vi "FrontEnd_Module.vi"() -> ()   [LabVIEW 2023]
uses:
  Controls/Select_Preference.ctl
  Controls/Coffee_Machine_Dispaly.ctl
  Controls/Queue_Operation_Select.ctl
  Controls/Coffee_Machine_Data.ctl
  Controls/Quantity_Data.ctl
  Controls/State_and_Data.ctl
  Controls/File_Operation_Select.ctl
  <vilib>/Utility/file.llb/Read Delimited Spreadsheet (string).vi
panel:
  out "Error_Out":errorcluster
  in  "Error_In":errorcluster
  in  "Power":bool
  out "Dispaly":T1 {"Dispenser" scale=0.0..80.0; "Chamber" scale=0.0..80.0}
  in  "Selector":T2 {"Select_Bevarage" scale=0.0..2.0}
  # "Coffee"
  # "Latte"
  # "Hot Water"
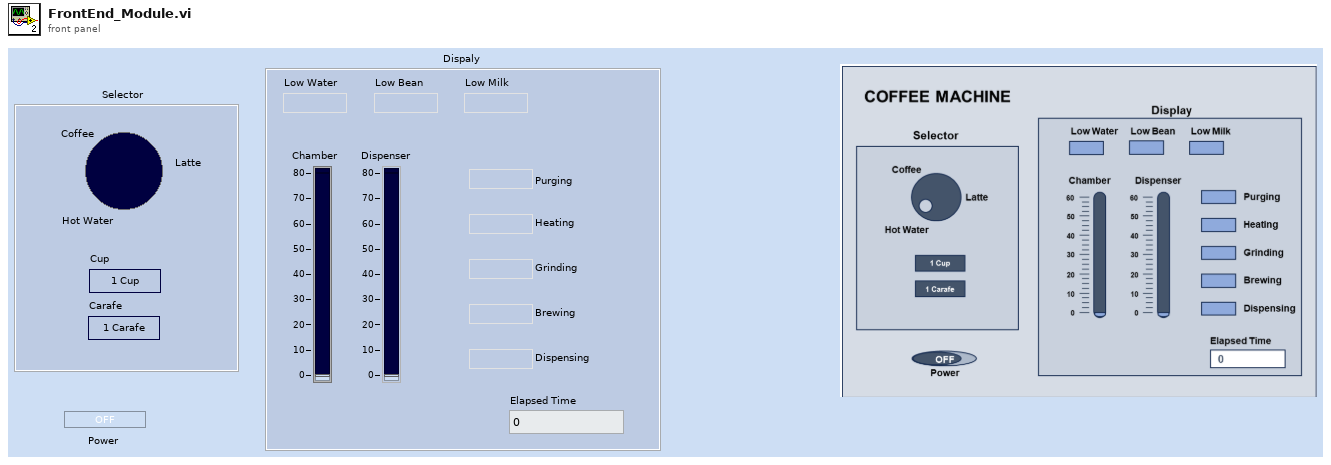
[diagram p1: front panel]
types:
  T1 = typedef "Coffee_Machine_Dispaly.ctl" = cluster{"Low_Water":bool, "Low_Bean":bool, "Low_Milk":bool, "Chamber":dbl, "Dispenser":dbl, "Purging":bool, "Heating":bool, "Grinding":bool, "Brewing":bool, "Dispensing":bool, "Elapsed_Time":dbl}
  T2 = typedef "Select_Preference.ctl" = cluster{"Select_Bevarage":i32, "Cup":bool, "Carafe":bool}
  T3 = typedef "State_and_Data.ctl" = cluster{"State":string, "Data":variant}
  T4 = typedef "Queue_Operation_Select.ctl" = enum16{"Obtain_Queue", "Enqueue", "Enqueue_First", "Enqueue_N", "Lossy_Enqueue", "Preview", "Queue_Status", "Dequeue", "Flush", "Release_Queue"}
  T5 = typedef "Coffee_Machine_Data.ctl" = cluster{"Backend_Data":T6, "Selector":T2, "Cup_Unit":dbl, "Carafe_Unit":dbl, "Ingreedient_File_PAth":path, "Process_Needed":string[], "Indredient_Needed":string[], "Time_Needed":string[], "State_and_Data":T3, "Chamber_Quantity":dbl, "Dispenser_Quantiry":dbl, "Dispaly":T1}
  T6 = typedef "Quantity_Data.ctl" = cluster{"Level":cluster{"Water_Level":dbl, "Bean_Level":dbl, "Milk_Level":dbl}, "Total_Cups":dbl}
  T7 = cluster{"Water_Level":dbl, "Bean_Level":dbl, "Milk_Level":dbl}
  T8 = typedef "File_Operation_Select.ctl" = enum16{"Open", "Read", "Write", "Close"}
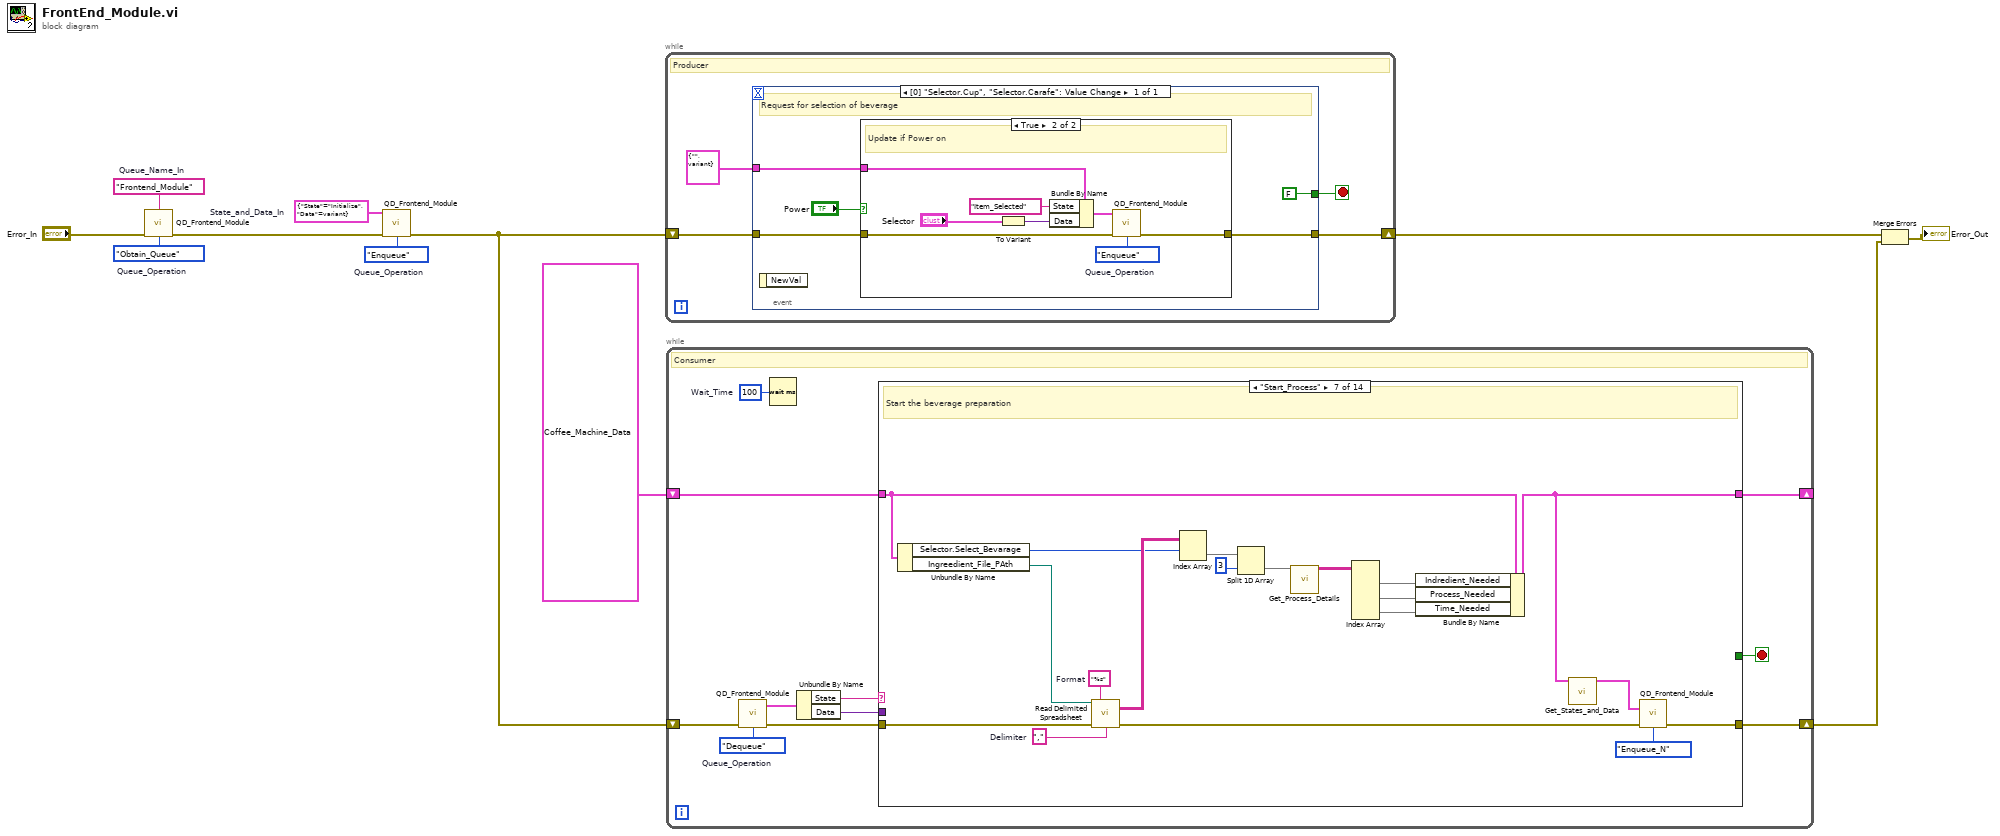
[diagram p0: block diagram]
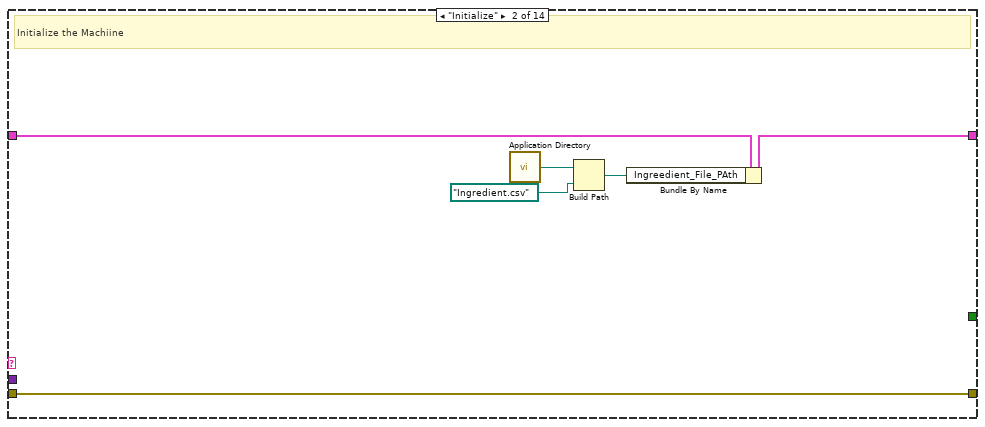
[diagram p3: hidden frame]
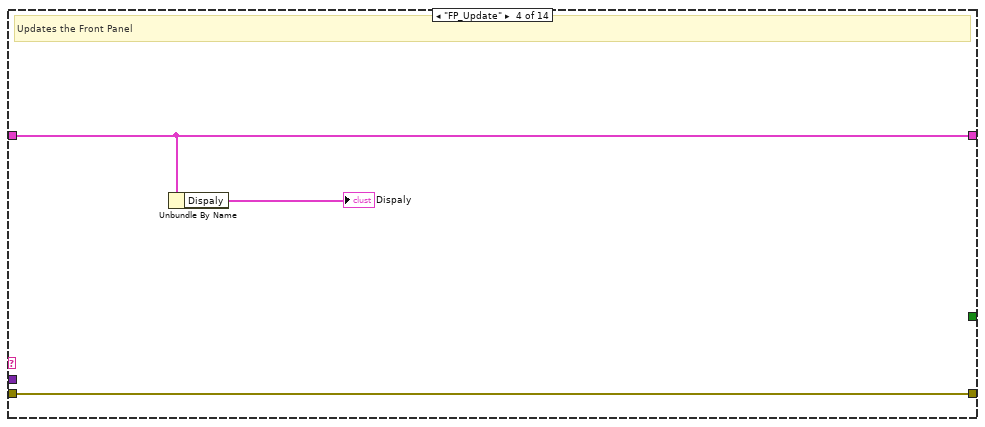
[diagram p5: hidden frame]
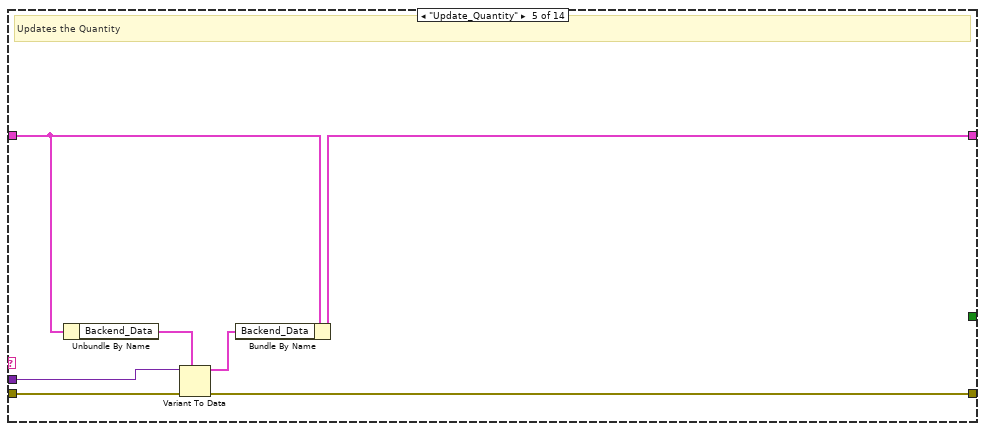
[diagram p6: hidden frame]
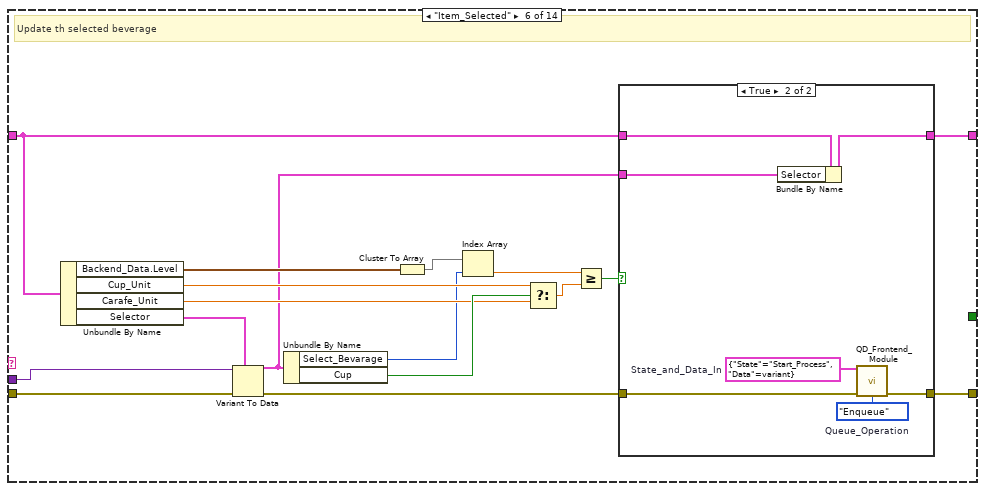
[diagram p7: hidden frame]
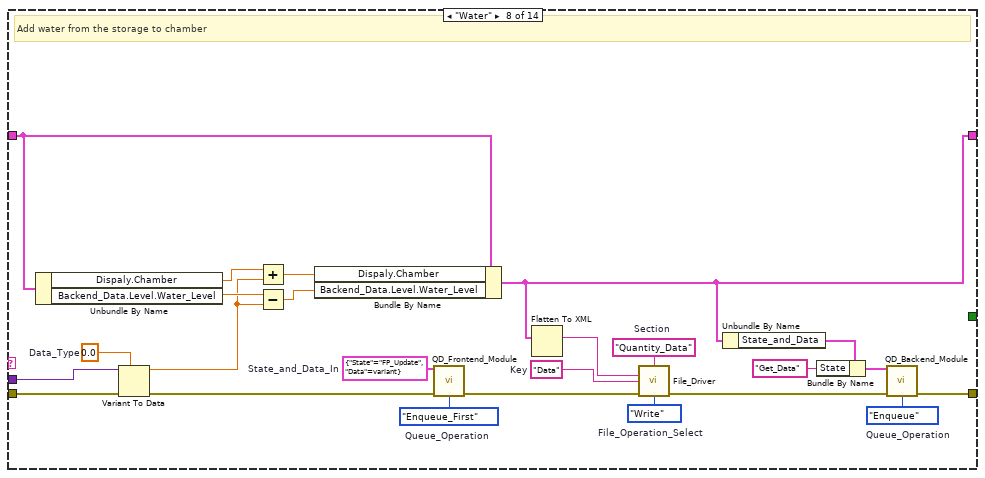
[diagram p9: hidden frame]
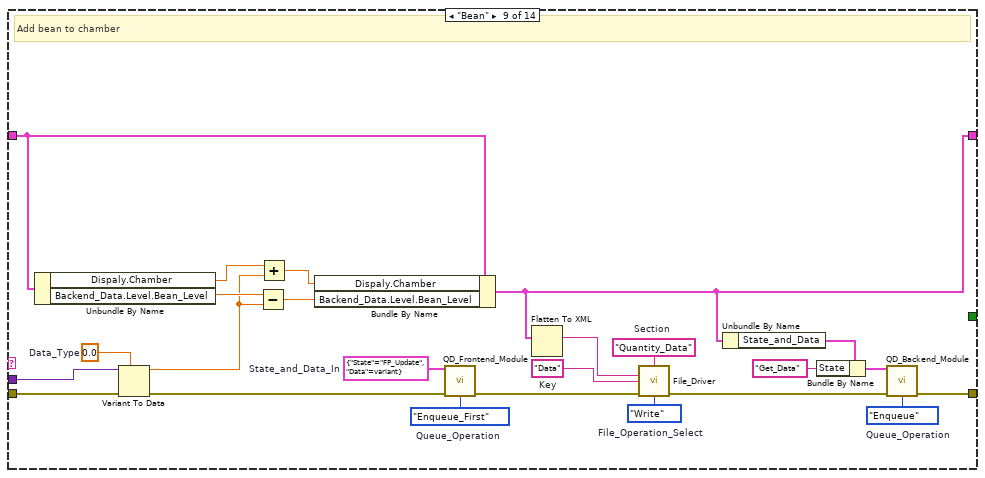
[diagram p10: hidden frame]
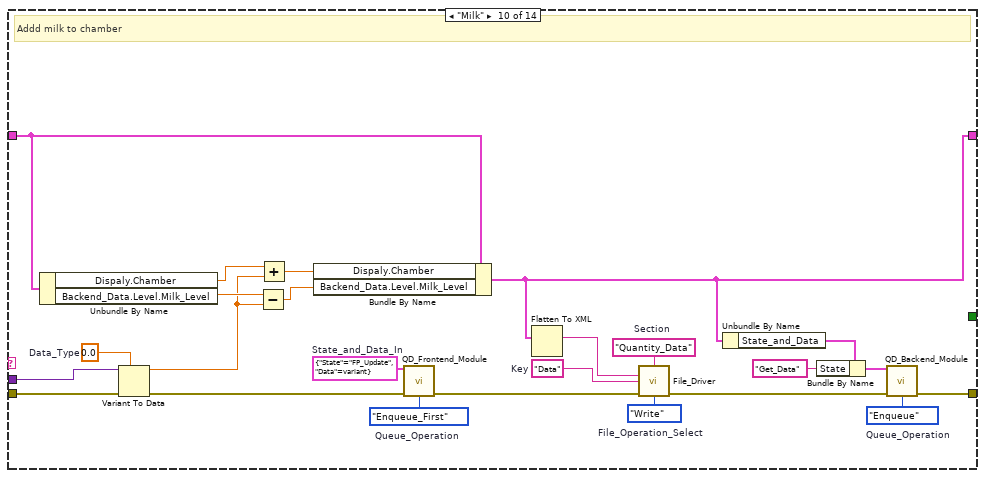
[diagram p11: hidden frame]
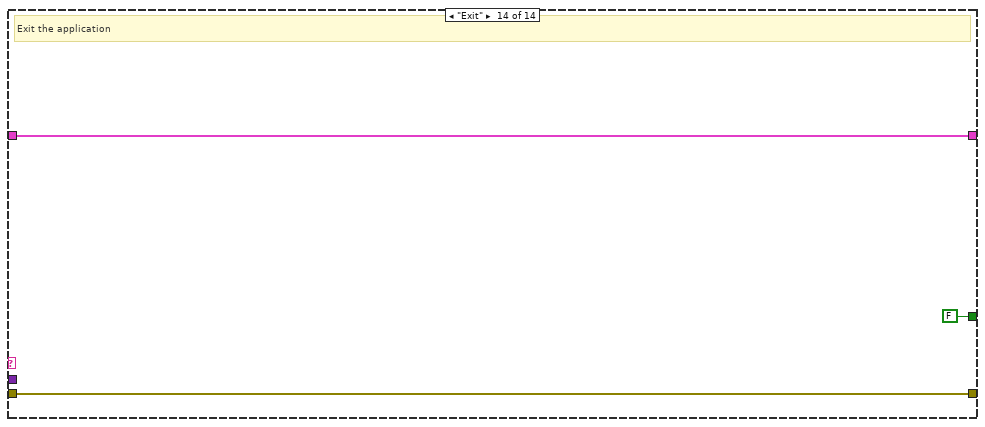
[diagram p15: hidden frame]
diagram:
  w1 = T3 {"State"="Initialize", "Data"=variant}  # State_and_Data_In
  w2 = Queue_Operation_Select."Enqueue"  # Queue_Operation
  w9 = "Frontend_Module"  # Queue_Name_In
  w10 = Queue_Operation_Select."Obtain_Queue"  # Queue_Operation
  n1 = call "QD_Frontend_Module.vi"("Queue_Name_In"=w9, "Error_In"="Error_In", "Queue_Operation"=w10) -> ("Error_Out"=w7:errorcluster)  [unwired: 10 in, 2 out]
  n2 = call "QD_Frontend_Module.vi"("State_and_Data_In"=w1, "Error_In"=w7, "Queue_Operation"=w2) -> ("Error_Out"=w3:errorcluster)  [unwired: 10 in, 2 out]
  n3 = while {
    shift-right: [w15] -> w8
    shift-left: w3 -> [w14]
    stop <- w12 stop-if-true
    # "Producer"
    n4 = event shown="[0] \"Selector.Cup\", \"Selector.Carafe\": Value Change" {
      selector: _ -> [_]
      dyn-events: _ -> [_]
      timeout: _ -> [_]
      tunnel: [w19] -> w15
      tunnel: w14 -> [w20]
      tunnel: T3 {"State"="", "Data"=variant} ("State_and_Data") -> [w18]
      tunnel: [FALSE] -> w12
      event Value Change {
        # "Request for selection of beverage"
        n5 = event-data() -> ()  [unwired: 1 in, 1 out]
        n6 = case shown="True" "Power" {
          tunnel: w20 -> [w21 w29]
          tunnel: [w21 w28] -> w19
          tunnel: w18 -> [_ w23]
          frame False {
          }
          frame True {
            w27 = Queue_Operation_Select."Enqueue"  # Queue_Operation
            # "Update if Power on"
            n7 = To Variant(anything="Selector") -> (Variant=w25:variant)
            n8 = Bundle By Name(cluster=w23, "State"="Item_Selected", "Data"=w25) -> (w24:T3)
            n9 = call "QD_Frontend_Module.vi"("State_and_Data_In"=w24, "Error_In"=w29, "Queue_Operation"=w27) -> ("Error_Out"=w28:errorcluster)  [unwired: 10 in, 2 out]
          }
        }
      }
    }
  }
  n10 = while {
    shift-right: [w32] -> _
    shift-left: T5 {"Backend_Data"={"Level"={"Water_Level"=0.0, "Bean_Level"=0.0, "Milk_Level"=0.0}, "Total_Cups"=0.0}, "Selector"={"Select_Bevarage"=0, "Cup"=FALSE, "Carafe"=FALSE}, "Cup_Unit"=5.0, "Carafe_Unit"=20.0, "Ingreedient_File_PAth"=path "", "Process_Needed"=[], "Indredient_Needed"=[], "Time_Needed"=[], "State_and_Data"={"State"="", "Data"=variant}, "Chamber_Quantity"=0.0, "Dispenser_Quantiry"=0.0, "Dispaly"={"Low_Water"=FALSE, "Low_Bean"=FALSE, "Low_Milk"=FALSE, "Chamber"=0.0, "Dispenser"=0.0, "Purging"=FALSE, "Heating"=FALSE, "Grinding"=FALSE, "Brewing"=FALSE, "Dispensing"=FALSE, "Elapsed_Time"=0.0}} -> [w33]
    shift-right: [w34] -> w4
    shift-left: w3 -> [w40]
    stop <- w31 stop-if-true
    w30 = u32 100  # Wait_Time
    w38 = Queue_Operation_Select."Dequeue"  # Queue_Operation
    # "Consumer"
    n11 = call "QD_Frontend_Module.vi"("Error_In"=w40, "Queue_Operation"=w38) -> ("State_and_Data_Out"=w37:T3, "Error_Out"=w39:errorcluster)  [unwired: 11 in, 1 out]
    n12 = Wait (ms)(milliseconds to wait=w30) -> ()  [unwired: 1 out]
    n13 = Unbundle By Name(w37) -> ("State"=w36:string, "Data"=w35:variant)
    n14 = case shown="\"Start_Process\"" w36 {
      tunnel: w39 -> [w42 w48 w50 w53 w60 w77 w105 w129 w153 w177 w179 w181 w183 w186]
      tunnel: w35 -> [_ _ _ _ w58 w76 _ w127 w152 w176 _ _ _ _]
      tunnel: [w42 w48 w50 w53 w59 w70 w93 w122 w147 w171 w179 w181 w183 w186] -> w34
      tunnel: w33 -> [w41 w47 w49 w52 w57 w63 w89 w125 w150 w174 w178 w180 w182 w185]
      tunnel: [w41 w46 w49 w52 w55 w64 w88 w115 w140 w164 w178 w180 w182 w185] -> w32
      tunnel: [_ _ _ _ _ _ _ _ _ _ _ _ _ FALSE] -> w31
      frame Default {
      }
      frame "Initialize" {
        # "Initialize the Machiine"
        n15 = call <vilib>:"Application Directory.vi"() -> ("Application Directory"=w44:path)
        n16 = Build Path(base path=w44, name or relative path=path "Ingredient.csv" ("Ingreedient_File_PAth")) -> (appended path=w45:path)
        n17 = Bundle By Name(cluster=w47, "Ingreedient_File_PAth"=w45) -> (w46:T5)
      }
      frame "Disable_and_Enable" {
        # "Disaable and enable"
      }
      frame "FP_Update" {
        # "Updates the Front Panel"
        n18 = Unbundle By Name(w52) -> ("Dispaly"=→"Dispaly":T1)
      }
      frame "Update_Quantity" {
        # "Updates the Quantity"
        n19 = Unbundle By Name(w57) -> ("Backend_Data"=w56:T6)
        n20 = Variant To Data(error in=w60, type=w56, Variant=w58) -> (data=w54:T6, error out=w59:errorcluster)
        n21 = Bundle By Name(cluster=w57, "Backend_Data"=w54) -> (w55:T5)
      }
      frame "Item_Selected" {
        # "Update th selected beverage"
        n22 = Unbundle By Name(w63) -> ("Backend_Data.Level"=w68:T7, "Cup_Unit"=w74:dbl, "Carafe_Unit"=w73:dbl, "Selector"=w62:T2)
        n23 = Variant To Data(error in=w77, type=w62, Variant=w76) -> (data=w61:T2, error out=w69:errorcluster)
        n24 = Unbundle By Name(w61) -> ("Select_Bevarage"=w66:i32, "Cup"=w75:bool)
        n25 = Cluster To Array(cluster=w68) -> (array=w67:dbl[])
        n26 = Index Array(array=w67, index=w66) -> (element=w65:dbl)
        n27 = Select(t=w74, s=w75, f=w73) -> (s? t:f=w71:dbl)
        n28 = Greater Or Equal?(x=w65, y=w71) -> (x >= y?=w72:bool)
        n29 = case shown="True" w72 {
          tunnel: [w78 w82] -> w70
          tunnel: w69 -> [w78 w86]
          tunnel: [w79 w84] -> w64
          tunnel: w63 -> [w79 w85]
          tunnel: w61 -> [_ w83]
          frame False {
          }
          frame True {
            w80 = T3 {"State"="Start_Process", "Data"=variant}  # State_and_Data_In
            w81 = Queue_Operation_Select."Enqueue"  # Queue_Operation
            n30 = Bundle By Name(cluster=w85, "Selector"=w83) -> (w84:T5)
            n31 = call "QD_Frontend_Module.vi"("State_and_Data_In"=w80, "Error_In"=w86, "Queue_Operation"=w81) -> ("Error_Out"=w82:errorcluster)  [unwired: 10 in, 2 out]
          }
        }
      }
      frame "Start_Process" {
        w102 = "%s"  # Format
        w103 = ","  # Delimiter
        # "Start the beverage preparation"
        n32 = Unbundle By Name(w89) -> ("Selector.Select_Bevarage"=w100:i32, "Ingreedient_File_PAth"=w87:path)
        n33 = call-poly <vilib>:"Read Delimited Spreadsheet.vi"("file path (dialog if empty)"=w87, "format (%s)"=w102, "error in (no error)"=w105, "delimiter (\\t)"=w103) -> ("all rows"=w101:string[][], "error out"=w104:errorcluster)  [unwired: 6 in, 4 out]
        n34 = Index Array(array=w101, index (row)=w100) -> (element=w99:string[])  [unwired: 1 in]
        n35 = Split 1D Array(array=w99, index=3) -> (second subarray=w97:string[])  [unwired: 1 out]
        n36 = call "Get_Process_Details.vi"("Process_Data"=w97) -> ("Needs"=w96:string[][])  [unwired: 14 in]
        n37 = Index Array(array=w96) -> (element #1=w91:string[], element #2=w95:string[], element #3=w94:string[])  [unwired: 6 in]
        n38 = Bundle By Name(cluster=w89, "Indredient_Needed"=w91, "Process_Needed"=w95, "Time_Needed"=w94) -> (w88:T5)
        n39 = call "Get_States_and_Data.vi"("Coffee_Machine_Data"=w88) -> ("States_and_Data"=w90:T3[])  [unwired: 14 in]
        n40 = call "QD_Frontend_Module.vi"("State_and_Data_N_In"=w90, "Error_In"=w104, "Queue_Operation"=Queue_Operation_Select."Enqueue_N") -> ("Error_Out"=w93:errorcluster)  [unwired: 10 in, 2 out]
      }
      frame "Water" {
        w106 = Queue_Operation_Select."Enqueue_First"  # Queue_Operation
        w107 = T3 {"State"="FP_Update", "Data"=variant}  # State_and_Data_In
        w112 = "Quantity_Data"  # Section
        w113 = "Data"  # Key
        w116 = File_Operation_Select."Write"  # File_Operation_Select
        w121 = Queue_Operation_Select."Enqueue"  # Queue_Operation
        w126 = 0.0  # Data_Type
        # "Add water from the storage to chamber"
        n41 = Unbundle By Name(w125) -> ("Dispaly.Chamber"=w109:dbl, "Backend_Data.Level.Water_Level"=w124:dbl)
        n42 = Variant To Data(error in=w129, type=w126, Variant=w127) -> (data=w110:dbl, error out=w128:errorcluster)
        n43 = Add(x=w109, y=w110) -> (x+y=w111:dbl)
        n44 = Subtract(x=w124, y=w110) -> (x-y=w123:dbl)
        n45 = Bundle By Name(cluster=w125, "Dispaly.Chamber"=w111, "Backend_Data.Level.Water_Level"=w123) -> (w115:T5)
        n46 = call "QD_Frontend_Module.vi"("State_and_Data_In"=w107, "Error_In"=w128, "Queue_Operation"=w106) -> ("Error_Out"=w108:errorcluster)  [unwired: 10 in, 2 out]
        n47 = Flatten To XML(6:w115) -> (2:w114:string)
        n48 = call "File_Driver.vi"("Section"=w112, "Data_In"=w114, "Key"=w113, "Error_In"=w108, "File_Operation_Select"=w116) -> ("Error_Out"=w117:errorcluster)  [unwired: 9 in, 1 out]
        n49 = Unbundle By Name(w115) -> ("State_and_Data"=w119:T3)
        n50 = Bundle By Name(cluster=w119, "State"="Get_Data") -> (w120:T3)
        n51 = call "QD_Backend_Module.vi"("State_and_Data_In"=w120, "Error_In"=w117, "Queue_Operation"=w121) -> ("Error_Out"=w122:errorcluster)  [unwired: 10 in, 2 out]
      }
      frame "Bean" {
        w135 = Queue_Operation_Select."Enqueue_First"  # Queue_Operation
        w136 = T3 {"State"="FP_Update", "Data"=variant}  # State_and_Data_In
        w137 = "Quantity_Data"  # Section
        w138 = "Data"  # Key
        w141 = File_Operation_Select."Write"  # File_Operation_Select
        w146 = Queue_Operation_Select."Enqueue"  # Queue_Operation
        w151 = 0.0  # Data_Type
        # "Add bean to chamber"
        n52 = Unbundle By Name(w150) -> ("Dispaly.Chamber"=w132:dbl, "Backend_Data.Level.Bean_Level"=w149:dbl)
        n53 = Variant To Data(error in=w153, type=w151, Variant=w152) -> (data=w131:dbl, error out=w134:errorcluster)
        n54 = Subtract(x=w149, y=w131) -> (x-y=w148:dbl)
        n55 = Add(x=w132, y=w131) -> (x+y=w130:dbl)
        n56 = Bundle By Name(cluster=w150, "Dispaly.Chamber"=w130, "Backend_Data.Level.Bean_Level"=w148) -> (w140:T5)
        n57 = call "QD_Frontend_Module.vi"("State_and_Data_In"=w136, "Error_In"=w134, "Queue_Operation"=w135) -> ("Error_Out"=w133:errorcluster)  [unwired: 10 in, 2 out]
        n58 = Flatten To XML(6:w140) -> (2:w139:string)
        n59 = call "File_Driver.vi"("Section"=w137, "Data_In"=w139, "Key"=w138, "Error_In"=w133, "File_Operation_Select"=w141) -> ("Error_Out"=w142:errorcluster)  [unwired: 9 in, 1 out]
        n60 = Unbundle By Name(w140) -> ("State_and_Data"=w144:T3)
        n61 = Bundle By Name(cluster=w144, "State"="Get_Data") -> (w145:T3)
        n62 = call "QD_Backend_Module.vi"("State_and_Data_In"=w145, "Error_In"=w142, "Queue_Operation"=w146) -> ("Error_Out"=w147:errorcluster)  [unwired: 10 in, 2 out]
      }
      frame "Milk" {
        w156 = Queue_Operation_Select."Enqueue_First"  # Queue_Operation
        w157 = T3 {"State"="FP_Update", "Data"=variant}  # State_and_Data_In
        w161 = "Quantity_Data"  # Section
        w162 = "Data"  # Key
        w165 = File_Operation_Select."Write"  # File_Operation_Select
        w170 = Queue_Operation_Select."Enqueue"  # Queue_Operation
        w175 = 0.0  # Data_Type
        # "Addd milk to chamber"
        n63 = Unbundle By Name(w174) -> ("Dispaly.Chamber"=w160:dbl, "Backend_Data.Level.Milk_Level"=w173:dbl)
        n64 = Variant To Data(error in=w177, type=w175, Variant=w176) -> (data=w159:dbl, error out=w155:errorcluster)
        n65 = Subtract(x=w173, y=w159) -> (x-y=w172:dbl)
        n66 = Add(x=w160, y=w159) -> (x+y=w158:dbl)
        n67 = Bundle By Name(cluster=w174, "Dispaly.Chamber"=w158, "Backend_Data.Level.Milk_Level"=w172) -> (w164:T5)
        n68 = call "QD_Frontend_Module.vi"("State_and_Data_In"=w157, "Error_In"=w155, "Queue_Operation"=w156) -> ("Error_Out"=w154:errorcluster)  [unwired: 10 in, 2 out]
        n69 = Flatten To XML(6:w164) -> (2:w163:string)
        n70 = call "File_Driver.vi"("Section"=w161, "Data_In"=w163, "Key"=w162, "Error_In"=w154, "File_Operation_Select"=w165) -> ("Error_Out"=w166:errorcluster)  [unwired: 9 in, 1 out]
        n71 = Unbundle By Name(w164) -> ("State_and_Data"=w168:T3)
        n72 = Bundle By Name(cluster=w168, "State"="Get_Data") -> (w169:T3)
        n73 = call "QD_Backend_Module.vi"("State_and_Data_In"=w169, "Error_In"=w166, "Queue_Operation"=w170) -> ("Error_Out"=w171:errorcluster)  [unwired: 10 in, 2 out]
      }
      frame "Preparing" {
        # "Start preparing the beverage"
      }
      frame "Error" {
        # "Handle the error"
      }
      frame "Request_Exit" {
        # "Request error analysis"
      }
      frame "Exit" {
        # "Exit the application"
      }
    }
  }
  n74 = Merge Errors(w8, w4) -> (→"Error_Out":errorcluster)
